vi "wt1600 config from file.vi"(8 "WT1600 Config ing":T1={"Wiring A (0: 1P2W)"=0, "Wiring B (0: 1P2W)"=0, "Wiring C (0: 1P2W)"=0, "V Range (12: 1000)"=12, "V Element (0: All)"=0, "A Element (0: All)"=0, "A Range (9: 5A)"=9, "A Sensor Ratio(mV/A) (10.0000) "=10.0, "Zero Cross Filter (0: OFF)"=0, "Line Filter (0: OFF)"=0, "PT Ratio (1.0000)"=1.0, "Scaling (F: OFF)"=FALSE, "CT Ratio (1.0000)"=1.0, "Scaling Factor (1.0000)"=1.0, "Filter Element (0: All)"=0, "Display Format (0: Numeric)"=0, "Normal Item Amount (1: 4)"=1, "Harmonics Item Amount (1: 4)"=1, "Average Type (0: OFF)"=0, "Average Count (2: 8)"=2, "A Range (9: 5A) 2"=9, "A Sensor Ratio(mV/A) (10.0000)  2"=10.0, "Zero Cross Filter (0: OFF) 2"=0, "Line Filter (0: OFF) 2"=0, "PT Ratio (1.0000) 2"=1.0, "Scaling (F: OFF) 2"=FALSE, "CT Ratio (1.0000) 2"=1.0, "Scaling Factor (1.0000) 2"=1.0, "CUT OFF FREQ"=0.0} {"Scaling Factor (1.0000) 2" min=0.0001 max=99999.9999 step=0.0001 format="%.4f"; "CT Ratio (1.0000) 2" min=0.0001 max=99999.9999 step=0.0001 format="%.4f"; "PT Ratio (1.0000) 2" min=0.0001 max=99999.9999 step=0.0001 format="%.4f"; "Line Filter (0: OFF) 2" items=["OFF", "500Hz", "5.5kHz"]; "Zero Cross Filter (0: OFF) 2" items=["OFF", "500Hz"]; "A Sensor Ratio(mV/A) (10.0000)  2" min=0.0001 max=99999.9999 step=0.0001 format="%.4f"; "A Range (9: 5A) 2" items=["AUTO", "10 mA", "20 mA", "50 mA", "100 mA", "200 mA", "500 mA", "1 A", "2 A", "5 A", "10 A", "20 A", "50 A", "S-AUTO", "50 mV", "100 mV", "250 mV", "500 mV", "1 V", "2.5 V", "5 V", "10 V"]; "Average Count (2: 8)" items=["2", "4", "8", "16", "32", "64", "128", "256"]; "Average Type (0: OFF)" items=["OFF", "Linear", "Exponent"]; "Harmonics Item Amount (1: 4)" items=["-", "4", "8", "16", "Single List", "Dual List", "Sigma List"]; "Normal Item Amount (1: 4)" items=["ALL", "4", "8", "16", "42", "78"]; "Display Format (0: Numeric)" items=["Numeric", "Wave", "Bar", "Vector", "Trend", "Numeric & Wave", "Numeric & Bar", "Numeric & Trend", "Wave & Bar", "Wave & Trend", "Bar & Trend", "Information"]; "Filter Element (0: All)" items=["All", "Element 1", "Element 2", "Element 3", "Element 4", "Element 5", "Element 6"]; "Scaling Factor (1.0000)" min=0.0001 max=99999.9999 step=0.0001 format="%.4f"; "CT Ratio (1.0000)" min=0.0001 max=99999.9999 step=0.0001 format="%.4f"; "PT Ratio (1.0000)" min=0.0001 max=99999.9999 step=0.0001 format="%.4f"; "Line Filter (0: OFF)" items=["OFF", "500Hz", "5.5kHz"]; "Zero Cross Filter (0: OFF)" items=["OFF", "500Hz"]; "A Sensor Ratio(mV/A) (10.0000)" min=0.0001 max=99999.9999 step=0.0001 format="%.4f"; "A Range (9: 5A)" items=["AUTO", "10 mA", "20 mA", "50 mA", "100 mA", "200 mA", "500 mA", "1 A", "2 A", "5 A", "10 A", "20 A", "50 A", "S-AUTO", "50 mV", "100 mV", "250 mV", "500 mV", "1 V", "2.5 V", "5 V", "10 V"]; "A Element (0: All)" items=["All", "Element 1", "Element 2", "Element 3", "Element 4", "Element 5", "Element 6"]; "V Element (0: All)" items=["All", "Element 1", "Element 2", "Element 3", "Element 4", "Element 5", "Element 6"]; "V Range (12: 1000)" items=["AUTO", "1.5", "3", "6", "10", "15", "30", "60", "100", "150", "300", "600", "1000"]; "Wiring C (0: 1P2W)" items=["1P2W", "1P3W", "3P3W", "3P4W", "3V3A", "NONE"]; "Wiring B (0: 1P2W)" items=["1P2W", "1P3W", "3P3W", "3P4W", "3V3A", "NONE"]; "Wiring A (0: 1P2W)" items=["1P2W", "1P3W", "3P3W", "3P4W", "3V3A"]}, 10 "leggi":bool, 11 "Path":string) -> (0 "output cluster":T1)   [LabVIEW 2019]
panel:
  out "Numeric":dbl
  out "Array":string[][](array[string])
  # "ON\nOFF"
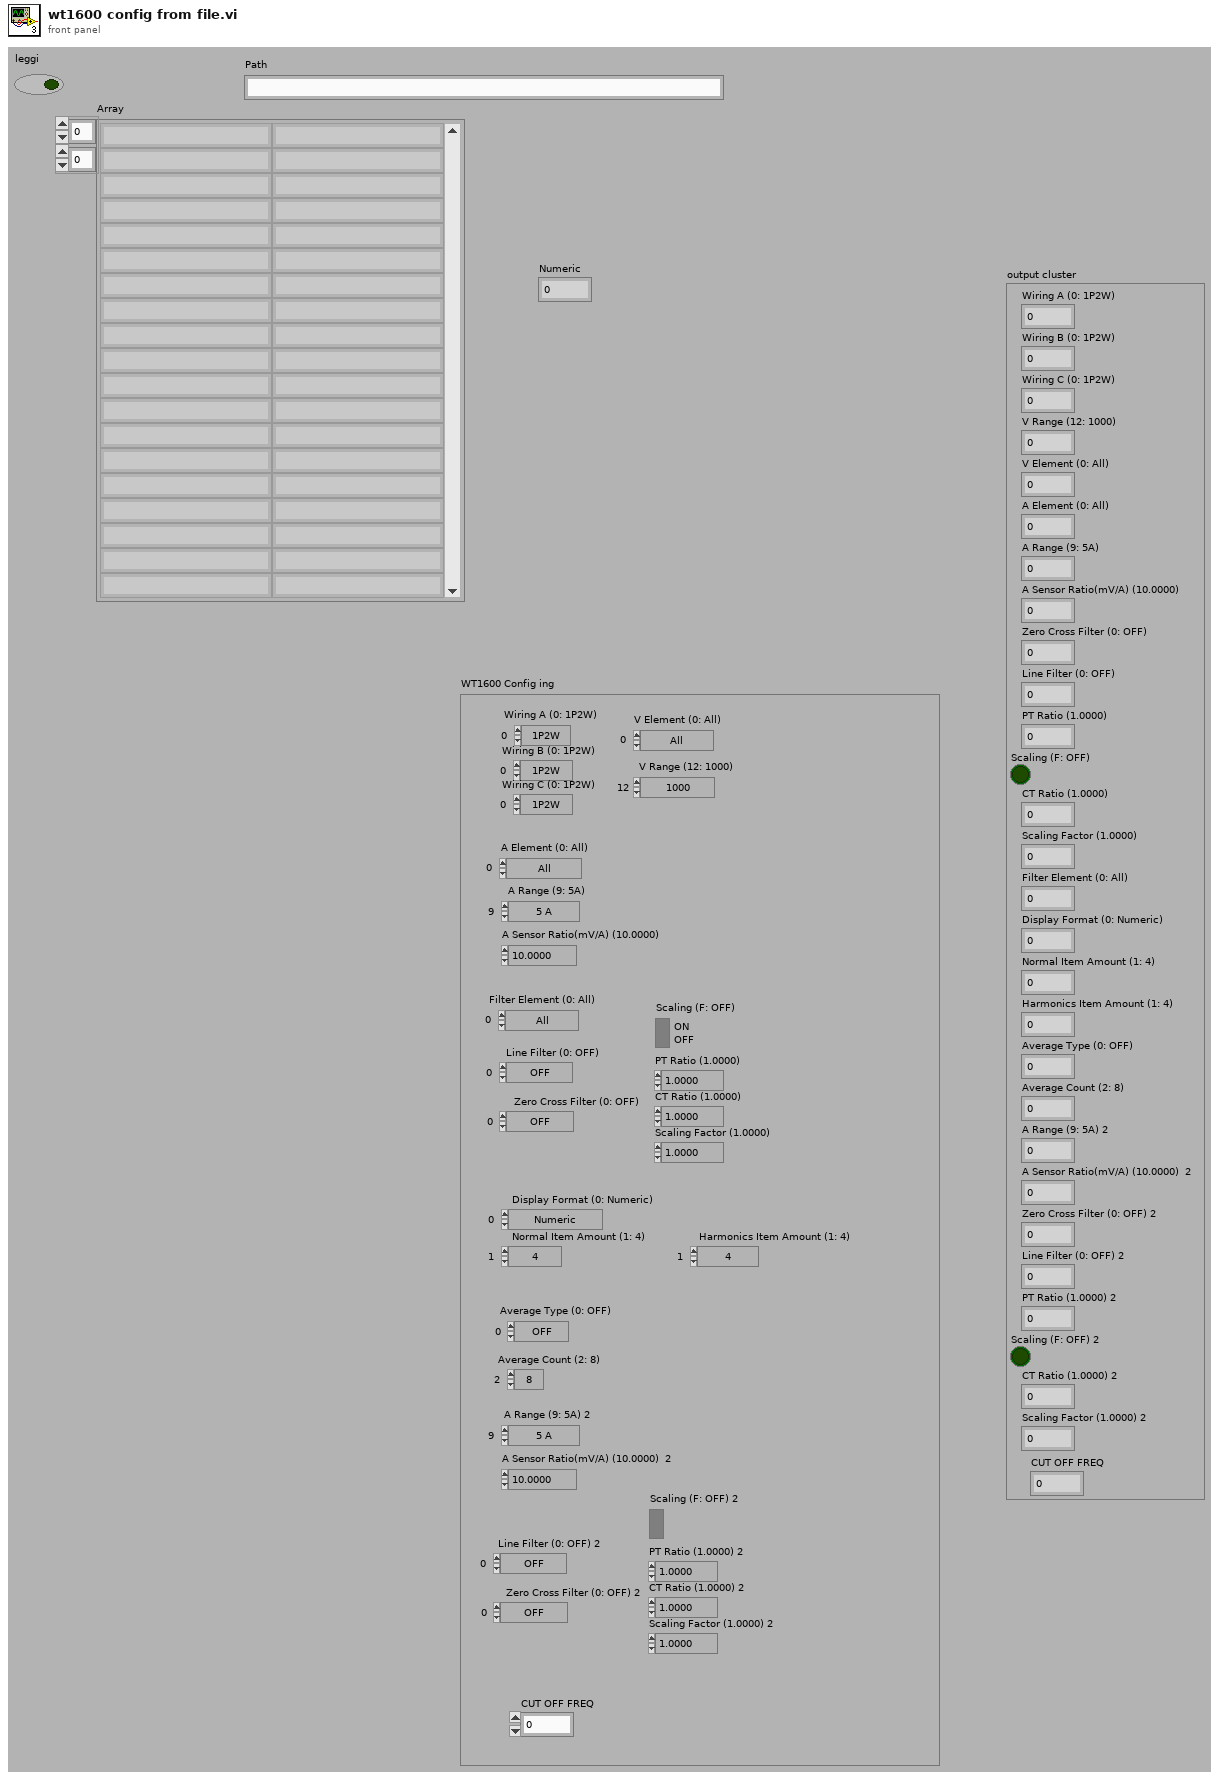
[diagram p1: front panel]
types:
  T1 = cluster{"Wiring A (0: 1P2W)":u16, "Wiring B (0: 1P2W)":u16, "Wiring C (0: 1P2W)":u16, "V Range (12: 1000)":u16, "V Element (0: All)":u16, "A Element (0: All)":u16, "A Range (9: 5A)":u16, "A Sensor Ratio(mV/A) (10.0000) ":dbl, "Zero Cross Filter (0: OFF)":u16, "Line Filter (0: OFF)":u16, "PT Ratio (1.0000)":dbl, "Scaling (F: OFF)":bool, "CT Ratio (1.0000)":dbl, "Scaling Factor (1.0000)":dbl, "Filter Element (0: All)":u16, "Display Format (0: Numeric)":u16, "Normal Item Amount (1: 4)":u16, "Harmonics Item Amount (1: 4)":u16, "Average Type (0: OFF)":u16, "Average Count (2: 8)":u16, "A Range (9: 5A) 2":u16, "A Sensor Ratio(mV/A) (10.0000)  2":dbl, "Zero Cross Filter (0: OFF) 2":u16, "Line Filter (0: OFF) 2":u16, "PT Ratio (1.0000) 2":dbl, "Scaling (F: OFF) 2":bool, "CT Ratio (1.0000) 2":dbl, "Scaling Factor (1.0000) 2":dbl, "CUT OFF FREQ":dbl}
  T2 = enum16{"open", "replace", "create", "open or create", "replace or create", "replace or create with confirmation"}
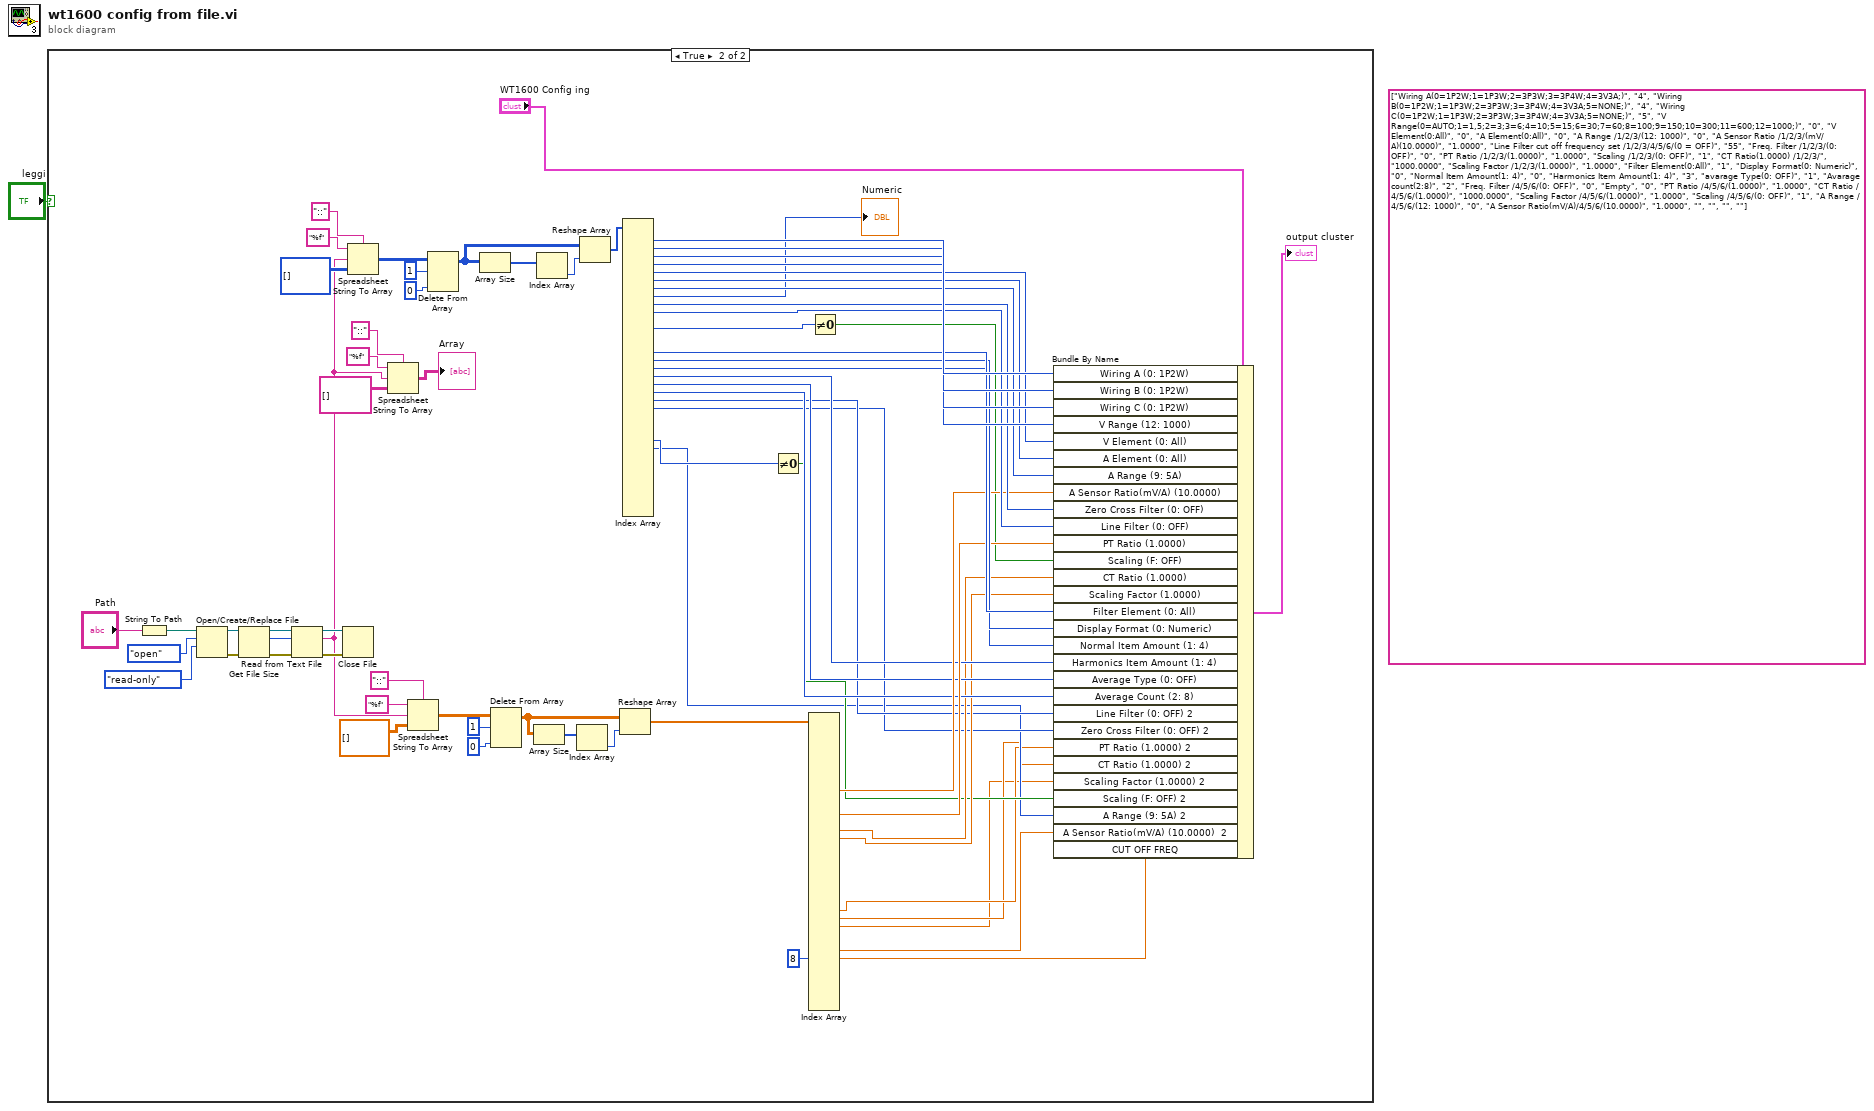
[diagram p0: block diagram]
diagram:
  (unwired) string[][] [["Wiring A(0=1P2W;1=1P3W;2=3P3W;3=3P4W;4=3V3A;)", "4"], ["Wiring B(0=1P2W;1=1P3W;2=3P3W;3=3P4W;4=3V3A;5=NONE;)", "4"], ["Wiring C(0=1P2W;1=1P3W;2=3P3W;3=3P4W;4=3V3A;5=NONE;)", "5"], ["V Range(0=AUTO;1=1,5;2=3;3=6;4=10;5=15;6=30;7=60;8=100;9=150;10=300;11=600;12=1000;)", "0"], ["V Element(0:All)", "0"], ["A Element(0:All)", "0"], ["A Range /1/2/3/(12: 1000)", "0"], ["A Sensor Ratio /1/2/3/(mV/A)(10.0000)", "1.0000"], ["Line Filter cut off frequency set /1/2/3/4/5/6/(0 = OFF)", "55"], ["Freq. Filter /1/2/3/(0: OFF)", "0"], ["PT Ratio /1/2/3/(1.0000)", "1.0000"], ["Scaling /1/2/3/(0: OFF)", "1"], ["CT Ratio(1.0000) /1/2/3/", "1000.0000"], ["Scaling Factor /1/2/3/(1.0000)", "1.0000"], ["Filter Element(0:All)", "1"], ["Display Format(0: Numeric)", "0"], ["Normal Item Amount(1: 4)", "0"], ["Harmonics Item Amount(1: 4)", "3"], ["avarage Type(0: OFF)", "1"], ["Avarage count(2:8)", "2"], ["Freq. Filter /4/5/6/(0: OFF)", "0"], ["Empty", "0"], ["PT Ratio /4/5/6/(1.0000)", "1.0000"], ["CT Ratio /4/5/6/(1.0000)", "1000.0000"], ["Scaling Factor /4/5/6/(1.0000)", "1.0000"], ["Scaling /4/5/6/(0: OFF)", "1"], ["A Range /4/5/6/(12: 1000)", "0"], ["A Sensor Ratio(mV/A)/4/5/6/(10.0000)", "1.0000"], ["", ""], ["", ""]] ("Array")
  n1 = case shown="True" "leggi" {
    frame False {
    }
    frame True {
      n2 = String To Path(string="Path") -> (path=w58:path)
      n3 = Open/Create/Replace File(file path (use dialog)=w58, operation (0:open)=T2."open", access (0:read/write)=enum16{"read/write", "read-only", "write-only"}."read-only") -> (refnum out=w63:refnum<file>, error out=w64:errorcluster)  [unwired: 1 in, 3 out]
      n4 = Get File Size(file=w63, error in=w64) -> (refnum out=w62:refnum<file>, size (in bytes)=w61:i64, 0:w60:errorcluster)
      n5 = Read from Text File(file (use dialog)=w62, count=w61, error in=w60) -> (refnum out=w67:refnum<file>, text=w22:string, error out=w66:errorcluster)  [unwired: 2 out]
      n6 = Close File(refnum=w67, error in=w66) -> ()  [unwired: 2 out]
      n7 = Spreadsheet String To Array(delimiter (Tab)="::", format string="%f", spreadsheet string=w22, array type (2D Dbl)=i32[][] [] ("Array")) -> (array=w70:i32[][])
      n8 = Spreadsheet String To Array(delimiter (Tab)="::", format string="%f", spreadsheet string=w22, array type (2D Dbl)=string[][] [] ("Array")) -> (array=→"Array":string[][])
      n9 = Spreadsheet String To Array(delimiter (Tab)="::", format string="%f", spreadsheet string=w22, array type (2D Dbl)=dbl[][] [] ("Array")) -> (array=w50:dbl[][])
      n10 = Delete From Array(array=w70, length=1, index (col)=0 ("disabled index (col)")) -> (array with subset deleted=w56:i32[][])  [unwired: 1 in, 1 out]
      n11 = Array Size(array=w56) -> (size(s)=w55:i32[])
      n12 = Delete From Array(array=w50, length=1, index (col)=0 ("disabled index (col)")) -> (array with subset deleted=w46:dbl[][])  [unwired: 1 in, 1 out]
      n13 = Array Size(array=w46) -> (size(s)=w45:i32[])
      n14 = Index Array(array=w55) -> (element=w54:i32)  [unwired: 1 in]
      n15 = Index Array(array=w45) -> (element=w44:i32)  [unwired: 1 in]
      n16 = Reshape Array(w56, w54) -> (w43:i32[])
      n17 = Reshape Array(w46, w44) -> (w42:dbl[])
      n18 = Index Array(array=w43) -> (element #1=w41:i32, element #2=w40:i32, element #3=w39:i32, element #4=w38:i32, element #5=w37:i32, element #6=w36:i32, element #7=w35:i32, element #8=→"Numeric":i32, element #9=w34:i32, element #10=w33:i32, element #12=w27:i32, element #15=w32:i32, element #16=w31:i32, element #17=w30:i32, element #18=w20:i32, element #19=w19:i32, element #20=w18:i32, element #21=w13:i32, element #22=w12:i32, element #26=w11:i32, element #27=w9:i32)  [unwired: 35 in, 14 out]
      n19 = Not Equal To 0?(x=w11) -> (x != 0?=w10:bool)
      n20 = Index Array(array=w42, index #29=8 ("index")) -> (element #8=w29:dbl, element #11=w28:dbl, element #13=w15:dbl, element #14=w14:dbl, element #23=w8:dbl, element #24=w7:dbl, element #25=w6:dbl, element #28=w5:dbl, element #29=w2:dbl)  [unwired: 34 in, 26 out]
      n21 = Not Equal To 0?(x=w27) -> (x != 0?=w26:bool)
      n22 = Bundle By Name(cluster="WT1600 Config ing", "Wiring A (0: 1P2W)"=w41, "Wiring B (0: 1P2W)"=w40, "Wiring C (0: 1P2W)"=w39, "V Range (12: 1000)"=w38, "V Element (0: All)"=w37, "A Element (0: All)"=w36, "A Range (9: 5A)"=w35, "A Sensor Ratio(mV/A) (10.0000)"=w29, "Zero Cross Filter (0: OFF)"=w34, "Line Filter (0: OFF)"=w33, "PT Ratio (1.0000)"=w28, "Scaling (F: OFF)"=w26, "CT Ratio (1.0000)"=w15, "Scaling Factor (1.0000)"=w14, "Filter Element (0: All)"=w32, "Display Format (0: Numeric)"=w31, "Normal Item Amount (1: 4)"=w30, "Harmonics Item Amount (1: 4)"=w20, "Average Type (0: OFF)"=w19, "Average Count (2: 8)"=w18, "Line Filter (0: OFF) 2"=w13, "Zero Cross Filter (0: OFF) 2"=w12, "PT Ratio (1.0000) 2"=w8, "CT Ratio (1.0000) 2"=w7, "Scaling Factor (1.0000) 2"=w6, "Scaling (F: OFF) 2"=w10, "A Range (9: 5A) 2"=w9, "A Sensor Ratio(mV/A) (10.0000)  2"=w5, "CUT OFF FREQ"=w2) -> (→"output cluster":T1)
    }
  }
